vi "Flipper Delay.vi"(7 "Shooting Delays":T1={"Unjam On"=100.0, "Unjam Off"=100.0, "Flipper On"=300.0, "Flipper Off"=200.0, "Hopper Up"=100.0}, 9 "RPM In Range":bool, 10 "Shoot Button":bool, 11 "Shoot Mode":bool) -> (1 "Unjam Out":bool, 3 "Flipper Out":bool)   [LabVIEW 2013]
uses:
  Flipper Mode.ctl
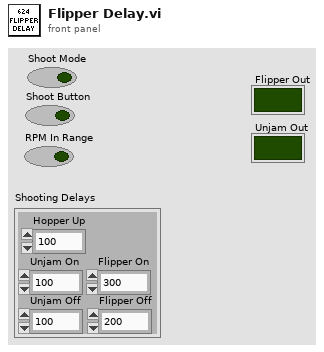
[diagram p1: front panel]
types:
  T1 = cluster{"Unjam On":dbl, "Unjam Off":dbl, "Flipper On":dbl, "Flipper Off":dbl, "Hopper Up":dbl}
  T2 = typedef "Flipper Mode.ctl" = enum16{"Wait for Shoot", "Hopper Up", "Wait for Button", "Unjam On", "Wait for RPM", "Flipper On", "Flipper Off", "Unjam Off"}
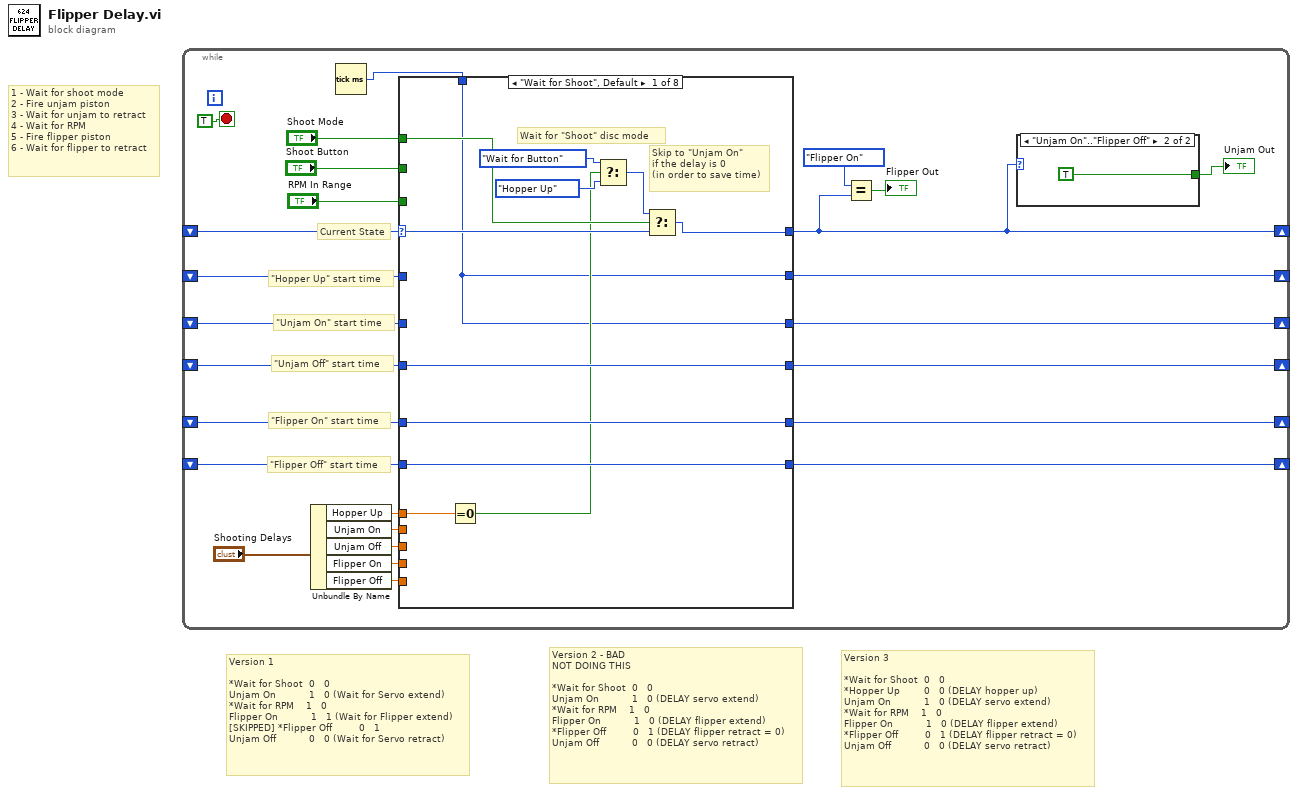
[diagram p0: block diagram]
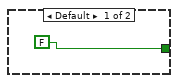
[diagram p2: hidden frame]
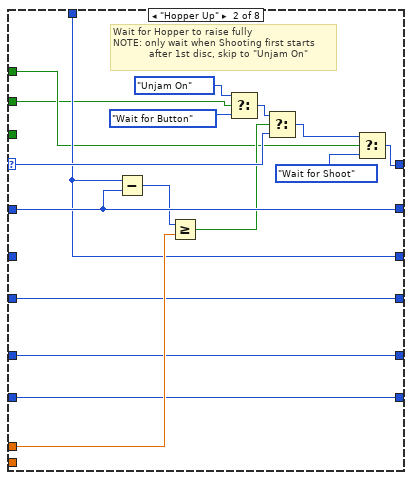
[diagram p3: hidden frame]
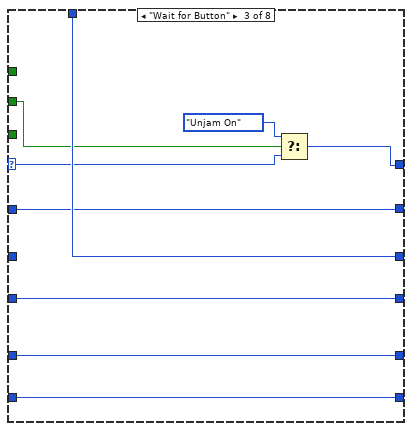
[diagram p4: hidden frame]
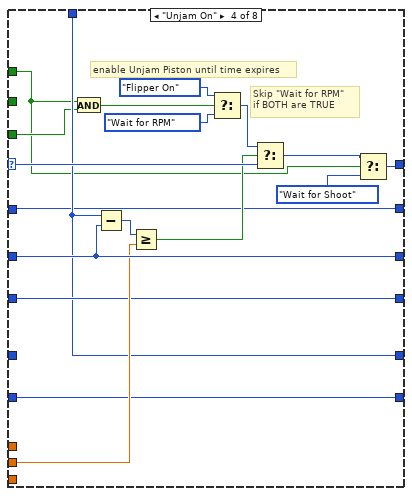
[diagram p5: hidden frame]
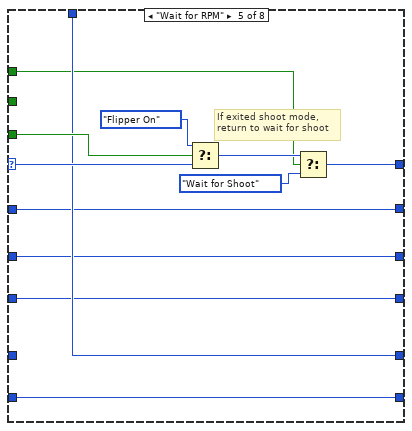
[diagram p6: hidden frame]
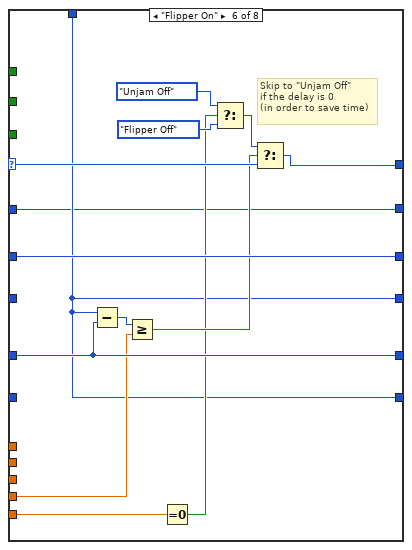
[diagram p7: hidden frame]
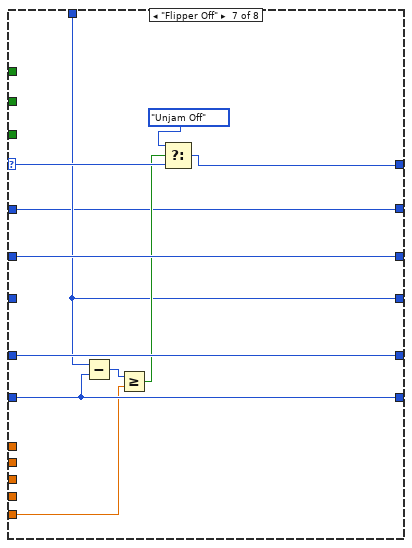
[diagram p8: hidden frame]
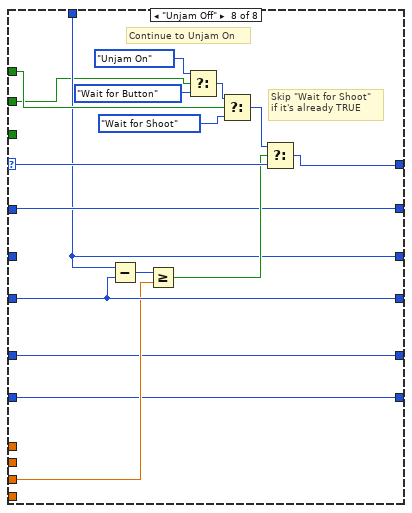
[diagram p9: hidden frame]
diagram:
  # "Version 3\n\n*Wait for Shoot  0   0\n*Hopper Up        0   0 (DELAY hopper up)\nUnjam On           1   0 (DELAY servo extend)\n*Wait for RPM    1   0\nFlipper On           1   0 (DELAY flipper extend)\n*Flipper Off         0   1 (DELAY flipper retract = 0)\nUnjam Off           0   0 (DELAY servo retract)"
  # "Version 2 - BAD\nNOT DOING THIS\n\n*Wait for Shoot  0   0\nUnjam On           1   0 (DELAY servo extend)\n*Wait for RPM    1   0\nFlipper On           1   0 (DELAY flipper extend)\n*Flipper Off         0   1 (DELAY flipper retract = 0)\nUnjam Off           0   0 (DELAY servo retract)"
  # "Version 1\n\n*Wait for Shoot  0   0\nUnjam On           1   0 (Wait for Servo extend)\n*Wait for RPM    1   0\nFlipper On           1   1 (Wait for Flipper extend)\n[SKIPPED] *Flipper Off         0   1\nUnjam Off           0   0 (Wait for Servo retract)"
  # "1 - Wait for shoot mode\n2 - Fire unjam piston\n3 - Wait for unjam to retract\n4 - Wait for RPM\n5 - Fire flipper piston \n6 - Wait for flipper to retract"
  n1 = while {
    shift-right: [w3] -> _
    shift-left: _ -> [w26]
    shift-right: [w23] -> _
    shift-left: _ -> [w22]
    shift-right: [w20] -> _
    shift-left: _ -> [w19]
    shift-right: [w13] -> _
    shift-left: _ -> [w12]
    shift-right: [w11] -> _
    shift-left: _ -> [w10]
    shift-right: [w5] -> _
    shift-left: _ -> [w4]
    stop <- TRUE stop-if-true
    # "\"Hopper Up\" start time"
    # "Current State"
    # "\"Flipper Off\" start time"
    # "\"Flipper On\" start time"
    # "\"Unjam Off\" start time"
    # "\"Unjam On\" start time"
    n2 = Unbundle By Name("Shooting Delays") -> ("Hopper Up"=w6:dbl, "Unjam On"=w15:dbl, "Unjam Off"=w14:dbl, "Flipper On"=w16:dbl, "Flipper Off"=w17:dbl)
    n3 = Tick Count (ms)() -> (millisecond timer value=w24:u32)
    n4 = case shown="\"Wait for Shoot\", Default" w26 {
      selector: w26 -> [w40 w57 w60 w84 w96 w110 w121 w138]
      tunnel: "RPM In Range" -> [_ _ _ w73 w95 _ _ _]
      tunnel: [w39 w47 w59 w68 w89 w109 w120 w131] -> w3
      tunnel: w24 -> [w29 w52 w66 w74 w94 w98 w112 w126]
      tunnel: [w29 w52 w66 w83 w93 w108 w119 w126] -> w23
      tunnel: w22 -> [_ _ _ w83 w93 w108 w119 _]
      tunnel: [w38 w49 w62 w79 w91 w98 w116 w132] -> w20
      tunnel: w19 -> [w38 w49 w62 w79 w91 _ w116 w132]
      tunnel: w17 -> [_ _ _ _ _ w101 w115 _]
      tunnel: w16 -> [_ _ _ _ _ w105 _ _]
      tunnel: "Shoot Mode" -> [w37 w45 _ w67 w88 _ _ w128]
      tunnel: w15 -> [_ _ _ w81 _ _ _ _]
      tunnel: w14 -> [_ _ _ _ _ _ _ w135]
      tunnel: [w36 w51 w64 w78 w92 w98 w112 w136] -> w13
      tunnel: w12 -> [w36 w51 w64 w78 w92 _ _ w136]
      tunnel: [w35 w50 w63 w74 w94 w106 w118 w133] -> w11
      tunnel: w10 -> [w35 w50 w63 _ _ w106 w118 w133]
      tunnel: w6 -> [w34 w54 _ _ _ _ _ _]
      tunnel: [w29 w56 w65 w71 w85 w97 w111 w127] -> w5
      tunnel: w4 -> [_ w56 w65 w71 w85 w97 w111 w127]
      tunnel: "Shoot Button" -> [_ w42 w61 _ _ _ _ w125]
      frame "Wait for Shoot", Default {
        # "Skip to \"Unjam On\"\nif the delay is 0\n(in order to save time)"
        # "Wait for \"Shoot\" disc mode"
        n5 = Equal To 0?(x=w34) -> (x = 0?=w30:bool)
        n6 = Select(t=Flipper_Mode."Wait for Button", s=w30, f=Flipper_Mode."Hopper Up" ("t")) -> (s? t:f=w33:T2)
        n7 = Select(t=w33, s=w37, f=w40) -> (s? t:f=w39:T2)
      }
      frame "Hopper Up" {
        # "Wait for Hopper to raise fully\nNOTE: only wait when Shooting first starts\n            after 1st disc, skip to \"Unjam On\""
        n8 = Subtract(x=w52, y=w56) -> (x-y=w55:u32)
        n9 = Greater Or Equal?(x=w55, y=w54) -> (x >= y?=w53:bool)
        n10 = Select(t=Flipper_Mode."Unjam On", s=w42, f=Flipper_Mode."Wait for Button" ("t")) -> (s? t:f=w43:T2)
        n11 = Select(t=w43, s=w53, f=w57) -> (s? t:f=w48:T2)
        n12 = Select(t=w48, s=w45, f=Flipper_Mode."Wait for Shoot") -> (s? t:f=w47:T2)
      }
      frame "Wait for Button" {
        n13 = Select(t=Flipper_Mode."Unjam On", s=w61, f=w60) -> (s? t:f=w59:T2)
      }
      frame "Unjam On" {
        # "Skip \"Wait for RPM\"\nif BOTH are TRUE"
        # "enable Unjam Piston until time expires"
        n14 = And(x=w67, y=w73) -> (x .and. y?=w72:bool)
        n15 = Subtract(x=w74, y=w83) -> (x-y=w82:u32)
        n16 = Greater Or Equal?(x=w82, y=w81) -> (x >= y?=w80:bool)
        n17 = Select(t=Flipper_Mode."Flipper On", s=w72, f=Flipper_Mode."Wait for RPM" ("t")) -> (s? t:f=w75:T2)
        n18 = Select(t=w75, s=w80, f=w84) -> (s? t:f=w70:T2)
        n19 = Select(t=w70, s=w67, f=Flipper_Mode."Wait for Shoot") -> (s? t:f=w68:T2)
      }
      frame "Wait for RPM" {
        # "If exited shoot mode,\nreturn to wait for shoot"
        n20 = Select(t=Flipper_Mode."Flipper On", s=w95, f=w96) -> (s? t:f=w90:T2)
        n21 = Select(t=w90, s=w88, f=Flipper_Mode."Wait for Shoot" ("t")) -> (s? t:f=w89:T2)
      }
      frame "Flipper On" {
        # "Skip to \"Unjam Off\"\nif the delay is 0\n(in order to save time)"
        n22 = Subtract(x=w98, y=w106) -> (x-y=w107:u32)
        n23 = Greater Or Equal?(x=w107, y=w105) -> (x >= y?=w104:bool)
        n24 = Equal To 0?(x=w101) -> (x = 0?=w100:bool)
        n25 = Select(t=Flipper_Mode."Unjam Off", s=w100, f=Flipper_Mode."Flipper Off" ("t")) -> (s? t:f=w99:T2)
        n26 = Select(t=w99, s=w104, f=w110) -> (s? t:f=w109:T2)
      }
      frame "Flipper Off" {
        n27 = Subtract(x=w112, y=w116) -> (x-y=w117:u32)
        n28 = Greater Or Equal?(x=w117, y=w115) -> (x >= y?=w114:bool)
        n29 = Select(t=Flipper_Mode."Unjam Off", s=w114, f=w121) -> (s? t:f=w120:T2)
      }
      frame "Unjam Off" {
        # "Continue to Unjam On"
        # "Skip \"Wait for Shoot\"\nif it's already TRUE"
        n30 = Subtract(x=w126, y=w136) -> (x-y=w137:u32)
        n31 = Greater Or Equal?(x=w137, y=w135) -> (x >= y?=w134:bool)
        n32 = Select(t=Flipper_Mode."Unjam On", s=w125, f=Flipper_Mode."Wait for Button" ("t")) -> (s? t:f=w122:T2)
        n33 = Select(t=w122, s=w128, f=Flipper_Mode."Wait for Shoot" ("t")) -> (s? t:f=w129:T2)
        n34 = Select(t=w129, s=w134, f=w138) -> (s? t:f=w131:T2)
      }
    }
    n35 = Equal?(x=Flipper_Mode."Flipper On" ("t"), y=w3) -> (x = y?=→"Flipper Out":bool)
    n36 = case shown="\"Unjam On\"..\"Flipper Off\"" w3 {
      tunnel: [FALSE TRUE] -> w9
      frame Default {
      }
      frame "Unjam On".."Flipper Off" {
      }
    }
    "Unjam Out" <- w9
  }
